vi "Convert to Tree Data.vi"(8 "error in (no error)":errorcluster, 11 "Data Cluster":T1) -> (0 "error out":errorcluster, 3 "Items out":T6(array[cluster]))   [LabVIEW 2020, in "Control Property Tree.lvlib"]
uses:
  Control Property Tree.lvlib
  Module Data--cluster.ctl
  Ctrl Properties Map Data.ctl
  Property array.ctl
  Selected Ctrls - List of Controls.ctl
  Selected Ctrls - List of Properties.ctl
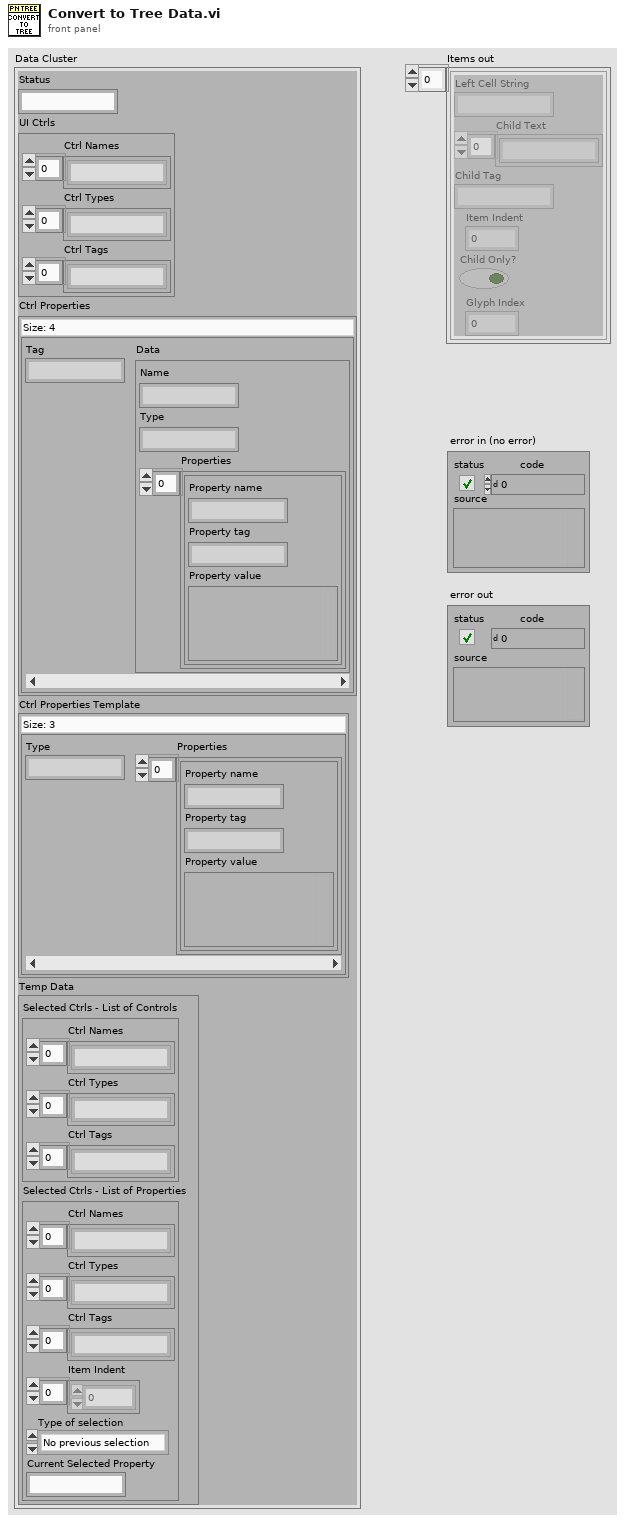
[diagram p1: front panel]
types:
  T1 = typedef "Control Property Tree.lvlib/Module Data--cluster.ctl" = cluster{"Status":string, "UI Ctrls":cluster{"Ctrl Names":string[], "Ctrl Types":string[], "Ctrl Tags":string[]}, "Ctrl Properties":map{string, T2}, "Ctrl Properties Template":map{string, T3}, "Temp Data":cluster{"Selected Ctrls - List of Controls":T4, "Selected Ctrls - List of Properties":T5}}
  T2 = typedef "Control Property Tree.lvlib/Ctrl Properties Map Data.ctl" = cluster{"Name":string, "Type":string, "Properties":T3}
  T3 = typedef "Control Property Tree.lvlib/Property array.ctl" = cluster{"Property name":string, "Property tag":string, "Property value":variant}[]
  T4 = typedef "Control Property Tree.lvlib/Selected Ctrls - List of Controls.ctl" = cluster{"Ctrl Names":string[], "Ctrl Types":string[], "Ctrl Tags":string[]}
  T5 = typedef "Control Property Tree.lvlib/Selected Ctrls - List of Properties.ctl" = cluster{"Ctrl Names":string[], "Ctrl Types":string[], "Ctrl Tags":string[], "Item Indent":i32[], "Type of selection":enum16{"No previous selection", "Control selected", "Property selected"}, "Current Selected Property":string}
  T6 = cluster{"Left Cell String":string, "Child Text":string[], "Child Tag":string, "Item Indent":i32, "Child Only?":bool, "Glyph Index":i32}[]
  T7 = cluster{"Left Cell String":string, "Child Text":string[], "Child Tag":string, "Item Indent":i32, "Child Only?":bool, "Glyph Index":i32}
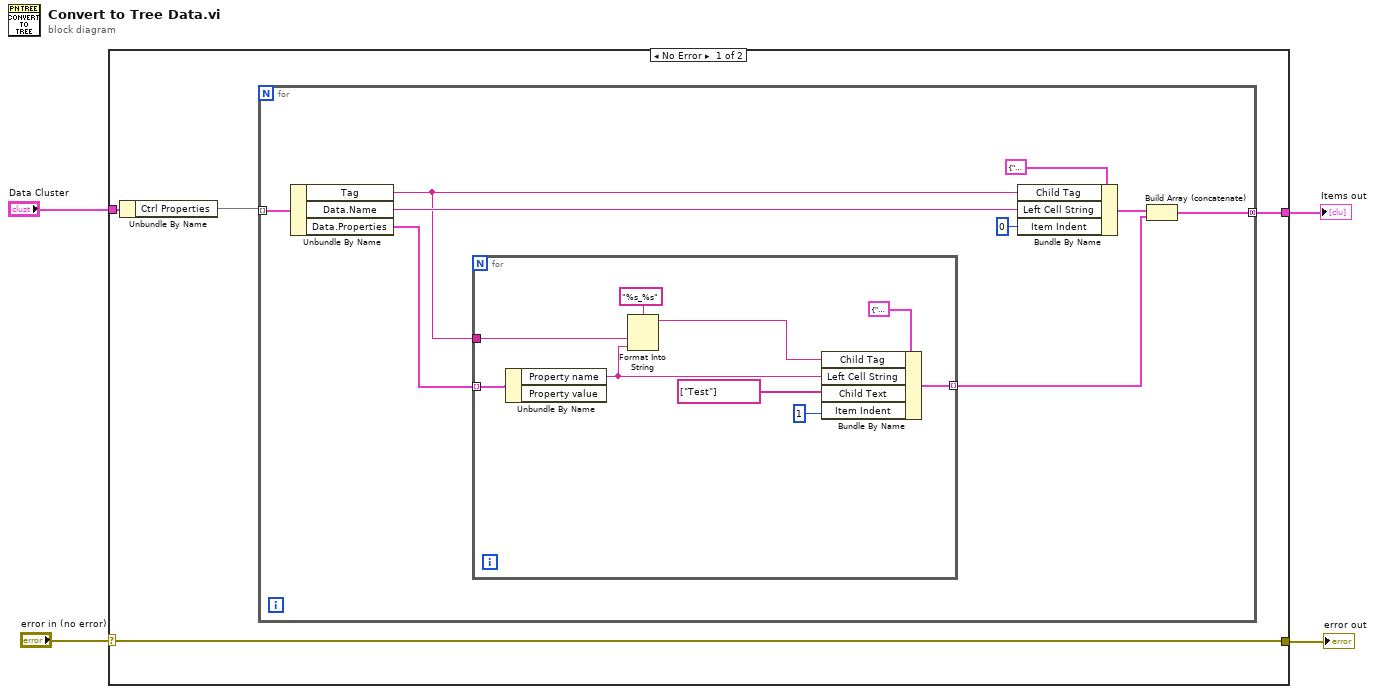
[diagram p0: block diagram]
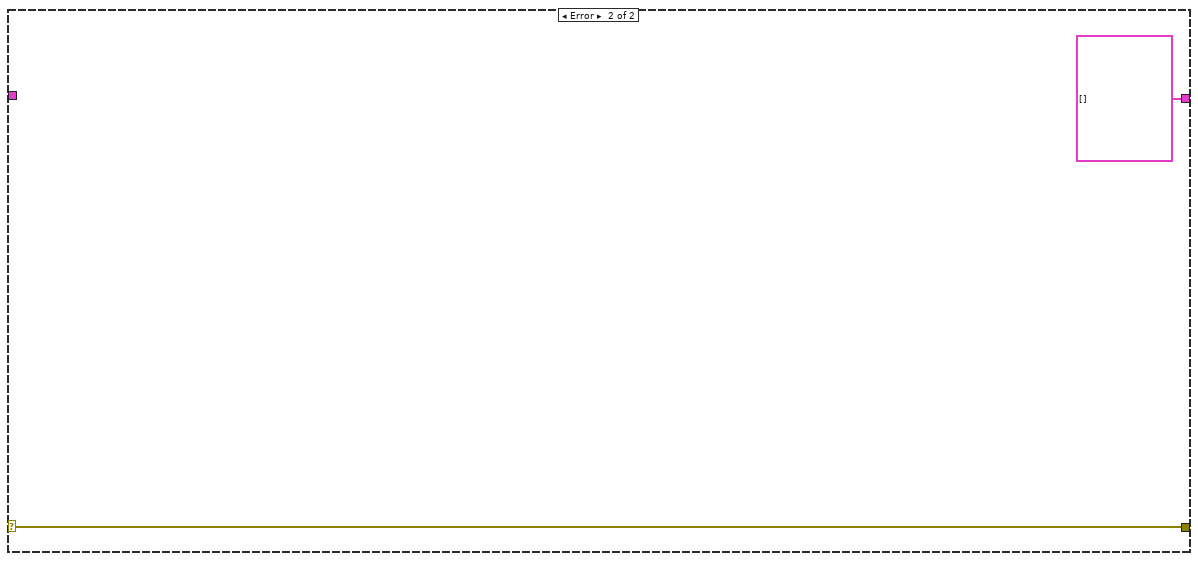
[diagram p2: hidden frame]
diagram:
  n1 = case shown="No Error" "error in (no error)" {
    selector: "error in (no error)" -> [w5 w28]
    tunnel: "Data Cluster" -> [w8 _]
    tunnel: [w6 T6 []] -> w3
    tunnel: [w5 w28] -> w1
    frame No Error {
      n2 = Unbundle By Name(w8) -> ("Ctrl Properties"=w7:map{string, T2})
      n3 = for {
        tunnel: w7 -> [w17] mode=indexing
        tunnel: [w9] -> w6 mode=concatenating
        n4 = Unbundle By Name(w17) -> ("Tag"=w12:string, "Data.Name"=w14:string, "Data.Properties"=w16:T3)
        n5 = for {
          tunnel: w16 -> [w26] mode=indexing
          tunnel: w12 -> [w23]
          tunnel: [w18] -> w10 mode=indexing
          n6 = Unbundle By Name(w26) -> ("Property name"=w22:string)  [unwired: 1 out]
          n7 = Format Into String(format string="%s_%s", w23, w22) -> (resulting string=w21:string)  [unwired: 2 in, 1 out]
          n8 = Bundle By Name(cluster=T7 {"Left Cell String"="", "Child Text"=[], "Child Tag"="", "Item Indent"=0, "Child Only?"=FALSE, "Glyph Index"=0} ("Item"), "Child Tag"=w21, "Left Cell String"=w22, "Child Text"=string[] ["Test"], "Item Indent"=1) -> (w18:T7)
        }
        n9 = Bundle By Name(cluster=T7 {"Left Cell String"="", "Child Text"=[], "Child Tag"="", "Item Indent"=0, "Child Only?"=FALSE, "Glyph Index"=0} ("Item"), "Child Tag"=w12, "Left Cell String"=w14, "Item Indent"=0) -> (w11:T7)
        n10 = Build Array (concatenate)(w11, w10) -> (w9:T6)
      }
    }
    frame Error {
    }
  }
  "Items out" <- w3
  "error out" <- w1
